vi "Agilent Ramp.vi"(7 "Frequency Hz":dbl=50.0, 8 "error in (no error)":errorcluster, 10 "VISA resource name":refnum<visa-resource-name>="GPIB0::10::INSTR", 11 "Vmax":dbl=2.0) -> (0 "error out":errorcluster)   [LabVIEW 2021]
uses:
  <instrlib>/Agilent 33XXX Series/Agilent 33XXX Series.lvlib
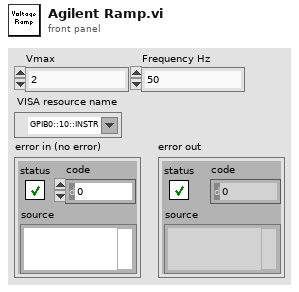
[diagram p1: front panel]
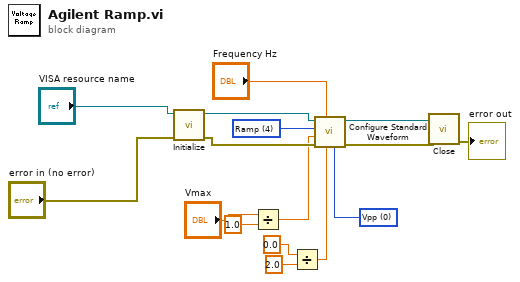
[diagram p0: block diagram]
diagram:
  w10 = u16 0 items=["Vpp", "Vrms", "dB"] ("Unit (0: Vpp)")
  w16 = u16 4 items=["DC", "Sine", "Square", "Triangle", "Ramp", "Pulse", "Noise", "Sinc", "Negative Ramp", "Exponential Rise", "Exponential Fall", "Cardiac"] ("Waveform Function (1: Sine)")
  n1 = call <instrlib>:"Initialize.vi"("error in (no error)"="error in (no error)", "VISA resource name"="VISA resource name") -> ("error out"=w13:errorcluster, "VISA resource name out"=w12:refnum<visa-resource-name>)  [unwired: 8 in]
  n2 = Divide(x="Vmax", y=1.0) -> (x/y=w7:dbl)
  n3 = Divide(x=0.0, y=2.0) -> (x/y=w5:dbl)
  n4 = call <instrlib>:"Configure Standard Waveform.vi"("Unit (0: Vpp)"=w10, "DC Offset (0.00 V)"=w5, "Frequency (1000 Hz)"="Frequency Hz", "error in (no error)"=w13, "Amplitude (1)"=w7, "Waveform Function (1: Sine)"=w16, "VISA resource name"=w12) -> ("error out"=w4:errorcluster, "VISA resource name out"=w3:refnum<visa-resource-name>)  [unwired: 3 in]
  n5 = call <instrlib>:"Close.vi"("error in (no error)"=w4, "VISA resource name"=w3) -> ("error out"=→"error out":errorcluster)  [unwired: 9 in]
